vi "Pack Four 16-bit to 64-bit (Single Tick)_Array.vi"(8 "Input Valid":bool=TRUE, 11 "Input":i16[](array[numeric])=[0, 0, 0, 0]) -> (0 "Output Valid":bool=TRUE, 3 "Output Data":u64)   [LabVIEW 2011]
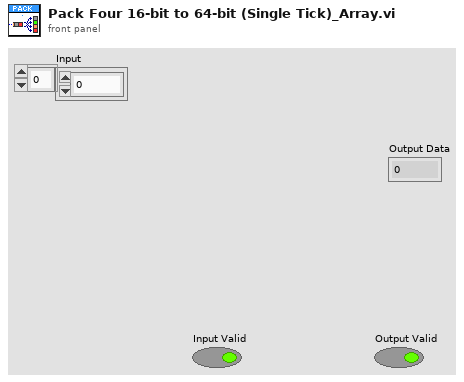
[diagram p1: front panel]
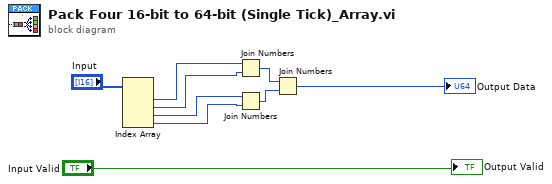
[diagram p0: block diagram]
diagram:
  n1 = Index Array(array="Input") -> (element #1=w5:i16, element #2=w4:i16, element #3=w3:i16, element #4=w2:i16)  [unwired: 4 in]
  n2 = Join Numbers(hi=w5, lo=w4) -> ((hi.lo)=w8:u32)
  n3 = Join Numbers(hi=w3, lo=w2) -> ((hi.lo)=w9:u32)
  n4 = Join Numbers(hi=w8, lo=w9) -> ((hi.lo)=→"Output Data":u64)
  "Output Valid" <- "Input Valid"
